vi "Simulate EPR peak.vi"() -> ()   [LabVIEW 2021]
uses:
  <vilib>/Analysis/4window.llb/Gaussian Window (DBL).vi
  0daa5ce1-9830-454e-ac7a-f6cbaae17fa9.vi
  <vilib>/Analysis/1siggen.llb/Ramp Pattern by Samples.vi
  <userlib>/_OpenG.lib/numeric/numeric.llb/Random Number Within Range - DBL__ogtk.vi
  <userlib>/_MGI/1D Array/MGI Calculate Array Differences/MGI Calculate Array Differences (DBL[]).vi
  <vilib>/Analysis/NI_AALBase.lvlib
  <vilib>/Analysis/NI_AALPro.lvlib
panel:
  out "Review Graph":cluster{"Array":dbl[], "Array":dbl[]}[](graph) caption="Header"
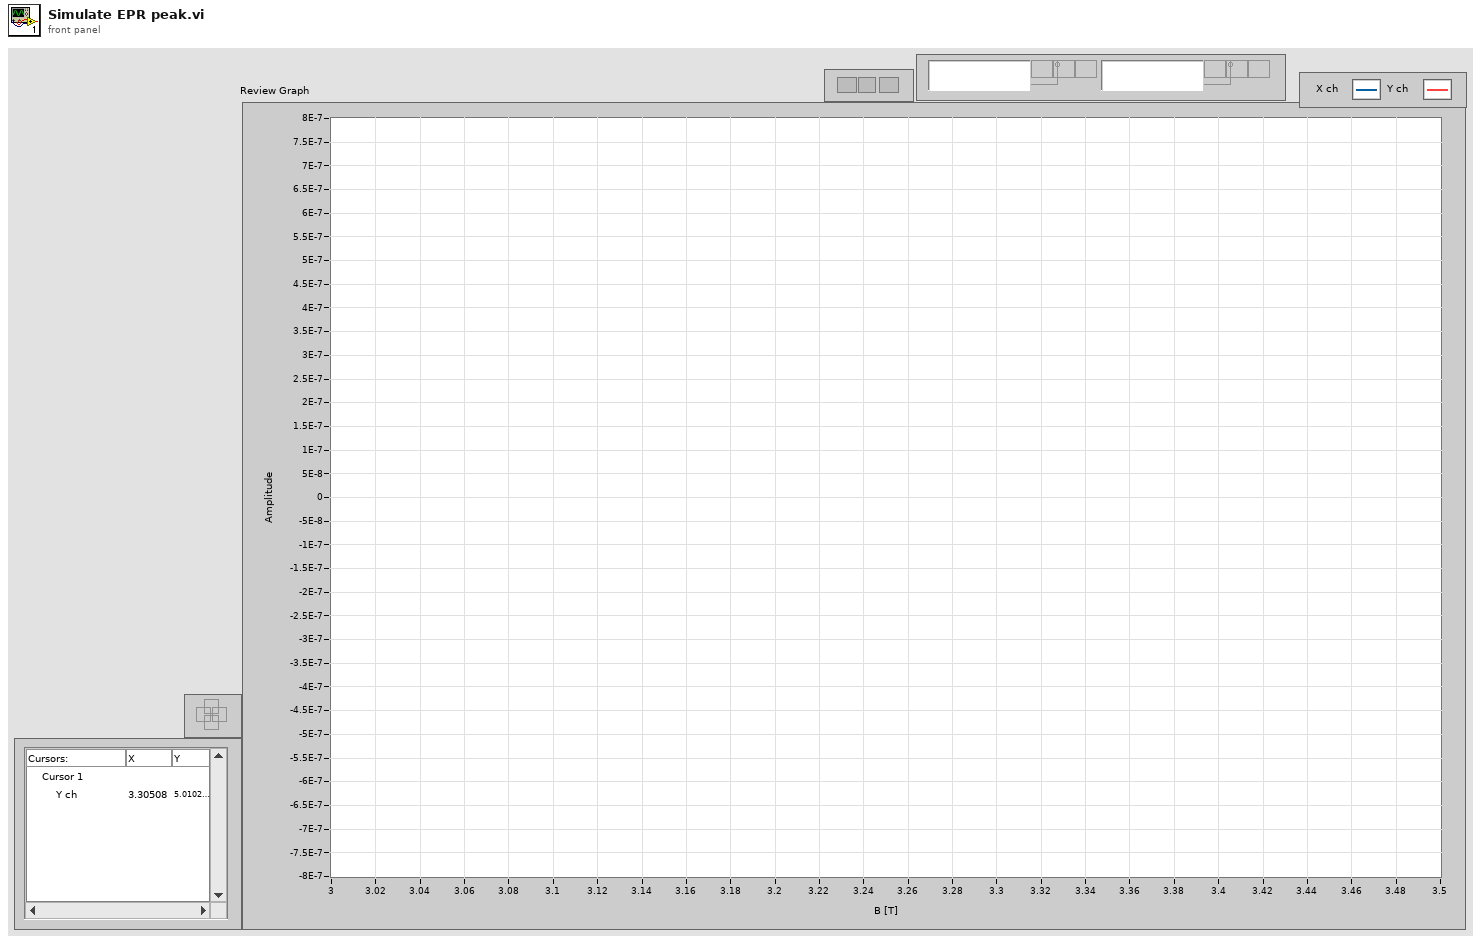
[diagram p1: front panel]
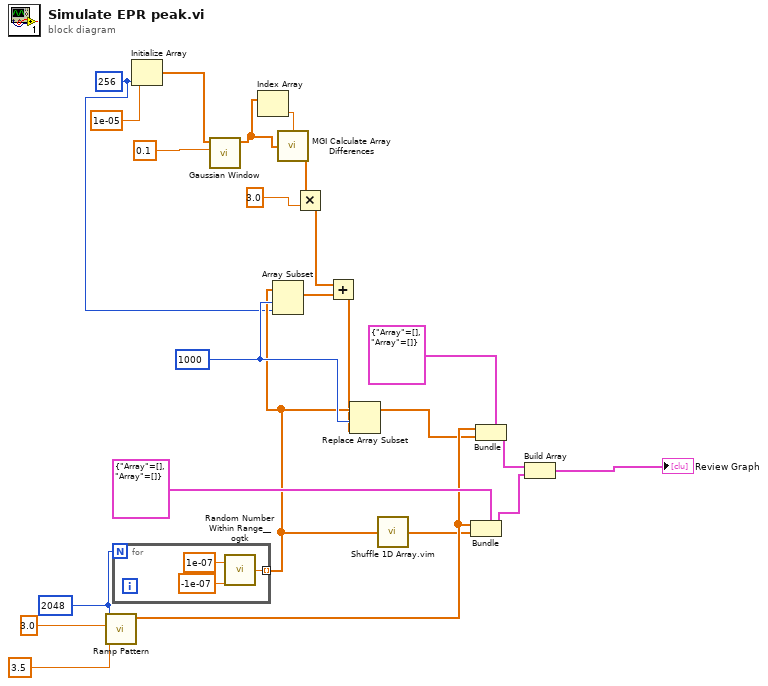
[diagram p0: block diagram]
diagram:
  w3 = 256 ("dimension size")
  w13 = 1000 ("index")
  w18 = 2048 ("samples")
  n1 = call-poly <vilib>:"Ramp Pattern.vi"("start"=3.0, "end"=3.5, "samples"=w18) -> ("Ramp Pattern"=w19:dbl[])  [unwired: 7 in, 1 out]
  n2 = for {
    N: w18 -> [_]
    tunnel: [w27] -> w12 mode=indexing
    n3 = call-poly <userlib>:"Random Number Within Range__ogtk.vi"("High"=1e-07, "Low"=-1e-07) -> ("Random Number"=w27:dbl)  [unwired: 3 in]
  }
  n4 = Initialize Array(1e-05 ("element"), w3) -> (w7:dbl[])
  n5 = call-poly <vilib>:"Gaussian Window.vi"("standard deviation"=0.1, "X"=w7) -> ("Windowed X"=w5:dbl[])  [unwired: 8 in, 1 out]
  n6 = Index Array(array=w5) -> (element=w6:dbl)  [unwired: 1 in]
  n7 = Array Subset(array=w12, index=w13, length=w3) -> (w10:dbl[])
  n8 = call-poly <userlib>:"MGI Calculate Array Differences.vi"("x(i)"=w5, "x(-1) (default 0)"=w6) -> ("y(i)=x(i)-x(i-1)"=w4:dbl[])
  n9 = Multiply(x=w4, y=3.0) -> (x*y=w2:dbl[])
  n10 = Add(x=w2, y=w10) -> (x+y=w11:dbl[])
  n11 = Replace Array Subset(array=w12, new element=w11, index=w13) -> (w16:dbl[])
  n12 = call "Shuffle 1D Array.vim"("array"=w12) -> ("shuffled array"=w17:dbl[])  [unwired: 4 in]
  n13 = Bundle(cluster=cluster{"Array":dbl[], "Array":dbl[]} {"Array"=[], "Array"=[]} ("Cluster"), "Array"=w19, "Array"=w17) -> (w21:cluster{"Array":dbl[], "Array":dbl[]})
  n14 = Bundle(cluster=cluster{"Array":dbl[], "Array":dbl[]} {"Array"=[], "Array"=[]} ("Cluster"), "Array"=w19, "Array"=w16) -> (w20:cluster{"Array":dbl[], "Array":dbl[]})
  n15 = Build Array(w20, w21) -> (→"Review Graph":cluster{"Array":dbl[], "Array":dbl[]}[])
